vi "createState.vi"(8 "error in (no error)":errorcluster, 10 "State:":T1=enum."EndingCycleState", 11 "IStateFactory in":refnum<class "IStateFactory.lvclass">) -> (0 "error out":errorcluster, 2 "State.lvclass":refnum<class "State.lvclass">, 3 "IStateFactory out":refnum<class "IStateFactory.lvclass">)   [LabVIEW 2013, in "IStateFactory.lvclass"]
uses:
  IStateFactory.lvclass
  Typedefs/StateSelector.ctl
  State/State.lvclass
  Typedefs/AITDTTypedefs.lvlib
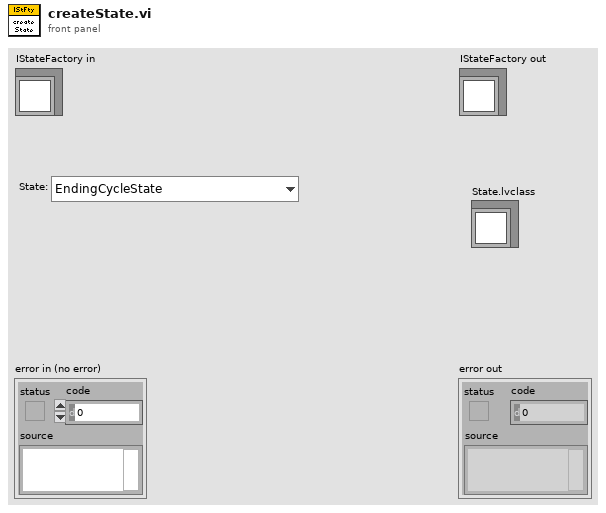
[diagram p1: front panel]
types:
  T1 = typedef "AITDTTypedefs.lvlib/StateSelector.ctl" = enum16{"AwaitingSetpointAcknowledgmentState", "EndingCycleState", "FaultState", "OffState", "PausingState", "RequestingNewSetpointState", "SamplingState", "SettlingState", "SoakingState", "StabilizingState", "StandbyState", "StoppedState", "TransitioningTemperatureState"}
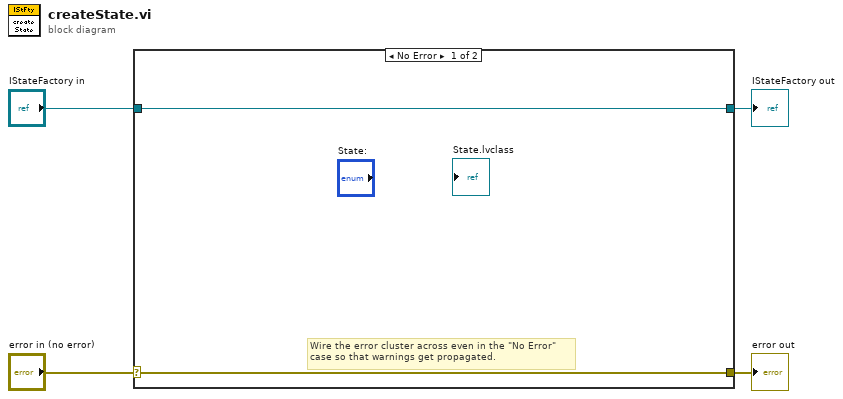
[diagram p0: block diagram]
diagram:
  n1 = case shown="No Error" "error in (no error)" {
    selector: "error in (no error)" -> [w5 w8]
    tunnel: [w5 w8] -> w3
    tunnel: [w6 w7] -> w1
    tunnel: "IStateFactory in" -> [w6 w7]
    frame No Error {
      # "Wire the error cluster across even in the \"No Error\"\ncase so that warnings get propagated."
    }
    frame Error {
    }
  }
  "error out" <- w3
  "IStateFactory out" <- w1
